vi "OnDrop.vi"(0 "XRef":T5, 1 "State In":T1) -> (14 "Reply":T3, 15 "Fatal Error Out":T2, 16 "State Out":T1)   [LabVIEW 2015, in "Index JSON Array.xnode"]
uses:
  Index JSON Array.xnode
  <vilib>/XNodeSupport/XNodeXNodeRef.ctl
  State.ctl
  <vilib>/XNodeSupport/XNodeStringArray.ctl
  <vilib>/XNodeSupport/XNodeString.ctl
  <vilib>/XNodeSupport/XNodeErrorCluster.ctl
  <vilib>/Utility/miscctls.llb/LVPointTypeDef.ctl
  class loader.vi
  <vilib>/XNodeSupport/NI_XNodeSupport.lvlib
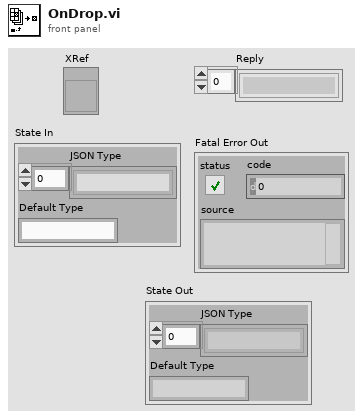
[diagram p1: front panel]
types:
  T1 = typedef "Index JSON Array.xnode/State.ctl" = cluster{"JSON Type":string[], "Default Type":string}
  T2 = typedef "NI_XNodeSupport.lvlib/XNodeErrorCluster.ctl" = errorcluster
  T3 = typedef "NI_XNodeSupport.lvlib/XNodeStringArray.ctl" = T4[]
  T4 = typedef "NI_XNodeSupport.lvlib/XNodeString.ctl" = string
  T5 = typedef "NI_XNodeSupport.lvlib/XNodeXNodeRef.ctl" = refnum<vi>
  T6 = typedef "LVPointTypeDef.ctl" = cluster{"Horizontal":i16, "Vertical":i16}
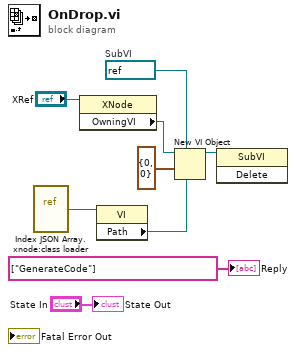
[diagram p0: block diagram]
diagram:
  w7 = refnum<vi> refnum  # SubVI
  n1 = vi-ref "Index JSON Array.xnode:class loader.vi"() -> (w2:refnum<vi>)
  n2 = property class="XNode"(reference="XRef") -> ("OwningVI"=w8:refnum<vi>)  [unwired: 1 in, 2 out]
  n3 = property class="VI"(reference=w2) -> ("Path"=w4:path)  [unwired: 1 in, 2 out]
  n4 = New VI Object(vi object class=w7, owner refnum=w8, position/next to=T6 {"Horizontal"=0, "Vertical"=0} ("location"), 6:w4) -> (object refnum=w5:refnum<vi>)  [unwired: 4 in, 1 out]
  n5 = invoke class="SubVI" method="Delete"(reference=w5) -> ()  [unwired: 2 in, 3 out]
  "Reply" <- T3 ["GenerateCode"] ("Reply")
  "State Out" <- "State In"
